vi "Fetch (NT Enum).vi"(7 "PV name":string, 8 "error in":errorcluster, 10 "default value":refnum<class "NT Enum.lvclass">, 11 "Server in":refnum<class "Server.lvclass">) -> (0 "error out":errorcluster, 1 "PV found?":bool, 2 "value":refnum<class "NT Enum.lvclass">, 3 "Server out":refnum<class "Server.lvclass">)   [LabVIEW 2020, in "PV Access.lvlib" / "PVA Server.lvlib" / "Server.lvclass"]
uses:
  Server.lvclass
  PV Data/NT Enum/NT Enum.lvclass
  C:/Users/eyw68381/source/repos/pvaccess-labview/labview/source/PV Data/NT Base/NT Base.lvclass
  PV Data/PV Data/PV Data.lvclass
  Source/Source.lvclass
  Server.lvclass/Server.ctl
  2ab69ff6-47d9-46ae-9252-a9f47d3d59e1.vi
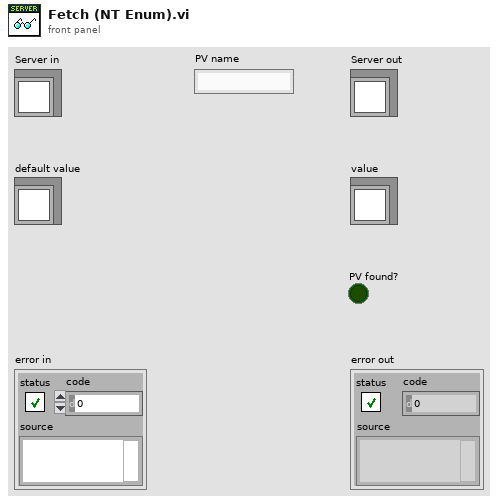
[diagram p1: front panel]
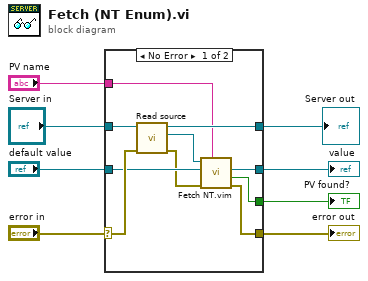
[diagram p0: block diagram]
diagram:
  n1 = case shown="No Error" "error in" {
    selector: "error in" -> [w18 w19]
    tunnel: [w11 w19] -> w4
    tunnel: "PV name" -> [w14 _]
    tunnel: "Server in" -> [w17 w21]
    tunnel: [w16 w21] -> w1
    tunnel: "default value" -> [w13 w20]
    tunnel: [w12 w20] -> w2
    tunnel: [w9 _] -> w3
    frame No Error {
      n2 = call "Read source.vi"("error in (no error)"=w18, "Server in"=w17) -> ("error out"=w10:errorcluster, "Source"=w15:refnum<class "Source.lvclass">, "Server out"=w16:refnum<class "Server.lvclass">)  [unwired: 7 in]
      n3 = call "Fetch NT.vim"("PV name"=w14, "error in"=w10, "default value"=w13, "Source in"=w15) -> ("error out"=w11:errorcluster, "PV found?"=w9:bool, "value"=w12:refnum<class "NT Enum.lvclass">)  [unwired: 4 in, 1 out]
    }
    frame Error {
    }
  }
  "Server out" <- w1
  "error out" <- w4
  "value" <- w2
  "PV found?" <- w3
